vi "Equações_Laminador.vi"(0 "DP_Lam [KPa]":dbl, 1 "B [(m³/h)/mmCA²]":dbl, 2 "C [(m³/h)/mmCA]":dbl, 3 "P* [KPa]":dbl, 4 "T* [K]":dbl, 5 "P_Bar [KPa]":dbl, 6 "P_Lam [KPa]":dbl, 7 "T_Lam [ºC]":dbl, 8 "Rho* [Kg/m³]":dbl, 9 "Mu* [Pa.s]":dbl, 10 "Diâmetro da tubulação [m]":dbl) -> (20 "DP_Lam [mmCA]":dbl, 21 "DP_Lam_max [mmCA]":bool, 22 "M_Lam [Kg/h]":dbl, 23 "Q* [m³/h]":dbl, 24 "Q_Lam [m³/h]":dbl, 25 "Jg [m/s]":dbl, 26 "Mu*/Mu_Lam":dbl, 27 "Rho_Nist/Rho*":dbl)   [LabVIEW 2019]
panel:
  out "Rho_Nist":dbl
  out "Erro_rel":dbl
  out "f0":dbl
  out "f1":dbl
  out "Delta_Mu [Pa.s]":dbl
  out "Mu100 [Pa.s]":dbl
  out "Mu_Lam [Pa.s]":dbl
  out "Rho_Lam [Kg/m³]":dbl
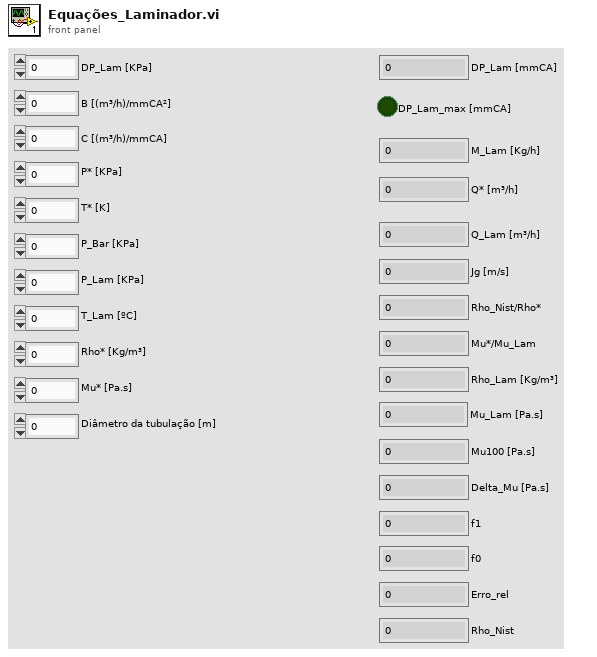
[diagram p1: front panel]
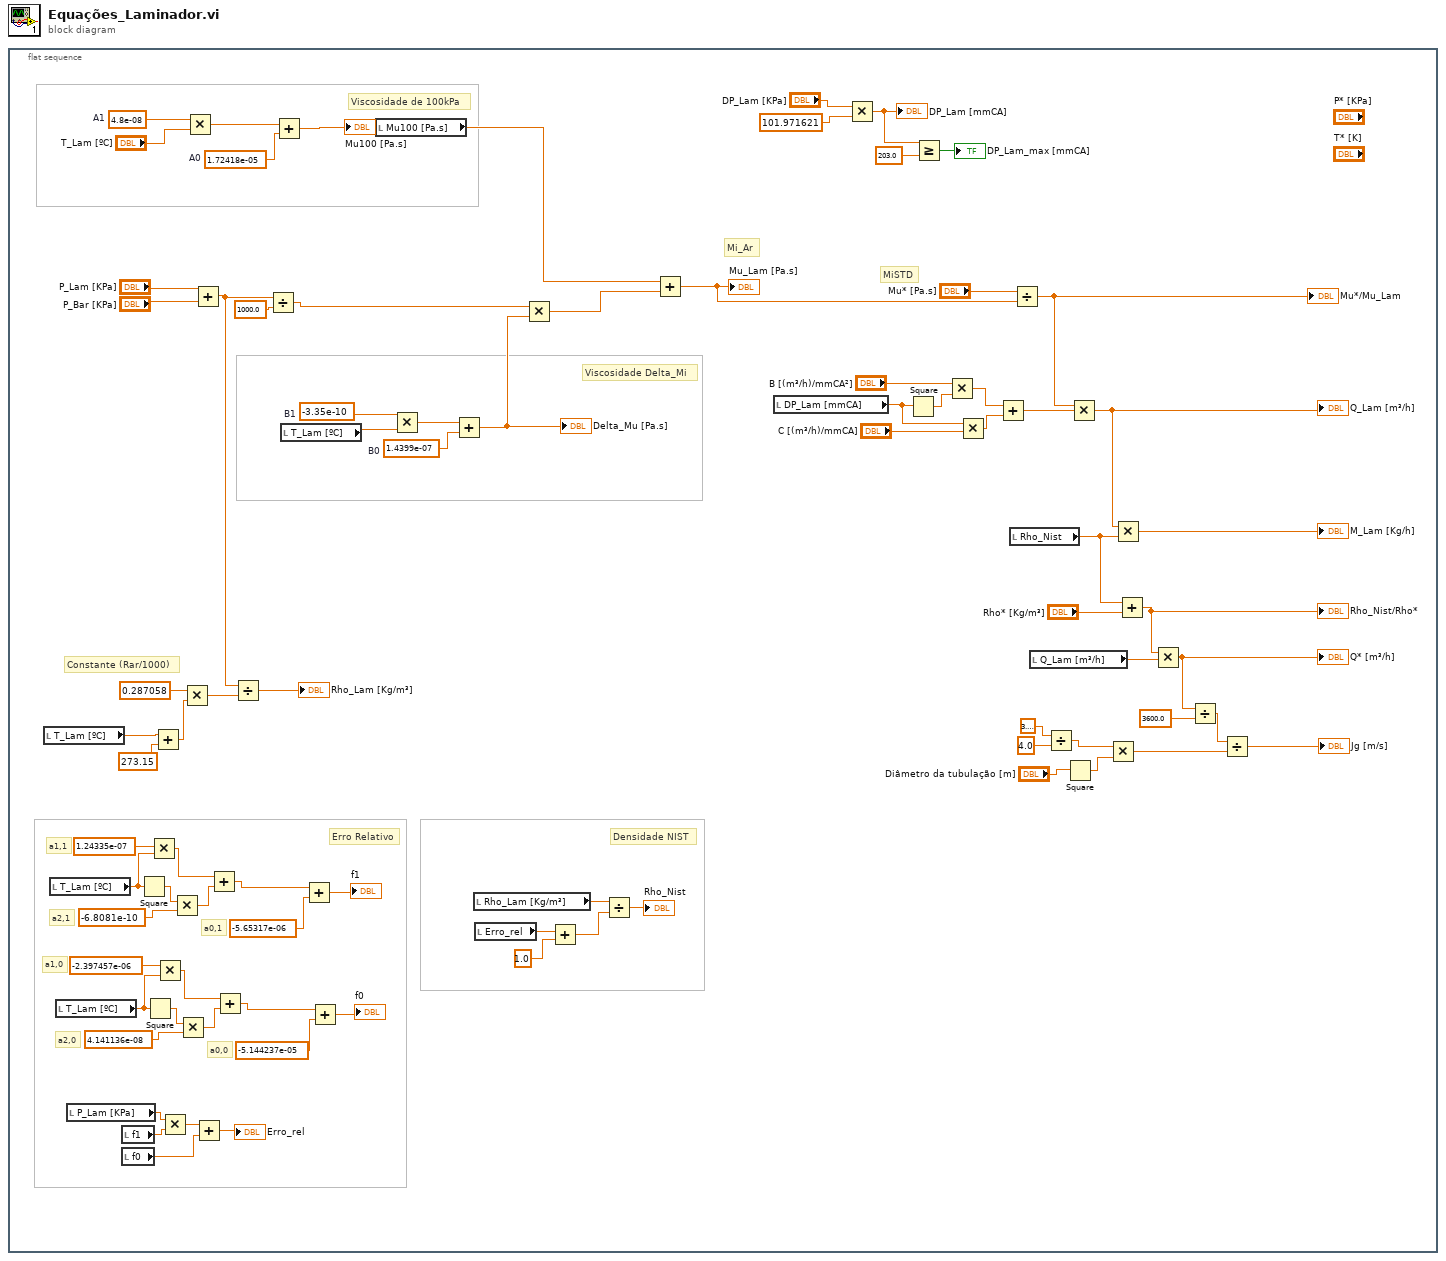
[diagram p0: block diagram]
diagram:
  n1 = flat-sequence {
    frame #0 {
      w79 = 1.4399e-07  # B0
      w81 = -3.35e-10  # B1
      w82 = 1.72418e-05  # A0
      w70 = 4.8e-08  # A1
      # "Densidade NIST"
      # "Erro Relativo"
      # "a0,0"
      # "a1,0"
      # "a2,0"
      # "a0,1"
      # "a1,1"
      # "a2,1"
      # "Constante (Rar/1000)"
      # "MiSTD"
      # "Viscosidade Delta_Mi"
      # "Mi_Ar"
      # "Viscosidade de 100kPa"
      n2 = local read "T_Lam [ºC]"() -> (w66:dbl)
      n3 = local read "T_Lam [ºC]"() -> (w28:dbl)
      n4 = local read "T_Lam [ºC]"() -> (w18:dbl)
      n5 = local read "P_Lam [KPa]"() -> (w13:dbl)
      n6 = local read "f1"() -> (w12:dbl)
      n7 = local read "f0"() -> (w10:dbl)
      n8 = Square(x=w28) -> (x^2=w31:dbl)
      n9 = Square(x=w18) -> (x^2=w15:dbl)
      n10 = Multiply(x=1.24335e-07, y=w28) -> (x*y=w29:dbl)
      n11 = Add(x=w66, y=273.15) -> (x+y=w73:dbl)
      n12 = Multiply(x=-2.397457e-06, y=w18) -> (x*y=w17:dbl)
      n13 = Multiply(x=w13, y=w12) -> (x*y=w11:dbl)
      n14 = Multiply(x=w31, y=-6.8081e-10) -> (x*y=w26:dbl)
      n15 = Multiply(x=w15, y=4.141136e-08) -> (x*y=w20:dbl)
      n16 = Multiply(x=0.287058, y=w73) -> (x*y=w72:dbl)
      n17 = Multiply(x=w70, y="T_Lam [ºC]") -> (x*y=w69:dbl)
      n18 = Add(x="P_Lam [KPa]", y="P_Bar [KPa]") -> (x+y=w63:dbl)
      n19 = Add(x=w11, y=w10) -> (x+y=→"Erro_rel":dbl)
      n20 = Add(x=w29, y=w26) -> (x+y=w25:dbl)
      n21 = Add(x=w17, y=w20) -> (x+y=w21:dbl)
      n22 = Divide(x=w63, y=w72) -> (x/y=→"Rho_Lam [Kg/m³]":dbl)
      n23 = Divide(x=w63, y=1000.0) -> (x/y=w3:dbl)
      n24 = Add(x=w69, y=w82) -> (x+y=→"Mu100 [Pa.s]":dbl)
      n25 = local read "T_Lam [ºC]"() -> (w67:dbl)
      n26 = Add(x=w25, y=-5.65317e-06) -> (x+y=→"f1":dbl)
      n27 = Add(x=w21, y=-5.144237e-05) -> (x+y=→"f0":dbl)
      n28 = local read "Mu100 [Pa.s]"() -> (w64:dbl)
      n29 = Multiply(x=w81, y=w67) -> (x*y=w80:dbl)
      n30 = Add(x=w80, y=w79) -> (x+y=w71:dbl)
      "Delta_Mu [Pa.s]" <- w71
      n31 = local read "Rho_Lam [Kg/m³]"() -> (w8:dbl)
      n32 = local read "Erro_rel"() -> (w6:dbl)
      n33 = Multiply(x=w3, y=w71) -> (x*y=w76:dbl)
      n34 = Add(x=w6, y=1.0) -> (x+y=w5:dbl)
      n35 = Divide(x=w8, y=w5) -> (x/y=→"Rho_Nist":dbl)
      n36 = Add(x=w64, y=w76) -> (x+y=w55:dbl)
      "Mu_Lam [Pa.s]" <- w55
      n37 = local read "DP_Lam [mmCA]"() -> (w52:dbl)
      n38 = Multiply(x="DP_Lam [KPa]", y=101.971621) -> (x*y=w58:dbl)
      "DP_Lam [mmCA]" <- w58
      n39 = Square(x=w52) -> (x^2=w53:dbl)
      n40 = Greater Or Equal?(x=w58, y=203.0) -> (x >= y?=→"DP_Lam_max [mmCA]":bool)
      n41 = Multiply(x="B [(m³/h)/mmCA²]", y=w53) -> (x*y=w50:dbl)
      n42 = Multiply(x=w52, y="C [(m³/h)/mmCA]") -> (x*y=w49:dbl)
      n43 = Add(x=w50, y=w49) -> (x+y=w47:dbl)
      n44 = local read "Rho_Nist"() -> (w2:dbl)
      n45 = Divide(x="Mu* [Pa.s]", y=w55) -> (x/y=w48:dbl)
      "Mu*/Mu_Lam" <- w48
      n46 = local read "Q_Lam [m³/h]"() -> (w42:dbl)
      n47 = Divide(x=3.141592653589793, y=4.0) -> (x/y=w41:dbl)
      n48 = Square(x="Diâmetro da tubulação [m]") -> (x^2=w40:dbl)
      n49 = Multiply(x=w48, y=w47) -> (x*y=w46:dbl)
      "Q_Lam [m³/h]" <- w46
      n50 = Multiply(x=w41, y=w40) -> (x*y=w33:dbl)
      n51 = Multiply(x=w46, y=w2) -> (x*y=→"M_Lam [Kg/h]":dbl)
      n52 = Add(x=w2, y="Rho* [Kg/m³]") -> (x+y=w43:dbl)
      "Rho_Nist/Rho*" <- w43
      n53 = Multiply(x=w43, y=w42) -> (x*y=w35:dbl)
      "Q* [m³/h]" <- w35
      n54 = Divide(x=w35, y=3600.0) -> (x/y=w34:dbl)
      n55 = Divide(x=w34, y=w33) -> (x/y=→"Jg [m/s]":dbl)
    }
  }
